vi "mxwScript_API_SetVal_NamedExternalNodeState.vi"(8 "error in (no error)":errorcluster, 10 "external node state":variant, 11 "external node name":string) -> (0 "error out":errorcluster, 3 "parameter":T1)   [LabVIEW 2020]
uses:
  codeGenAPISupport.llb/cgAPI_mxwScript_Parameter.ctl
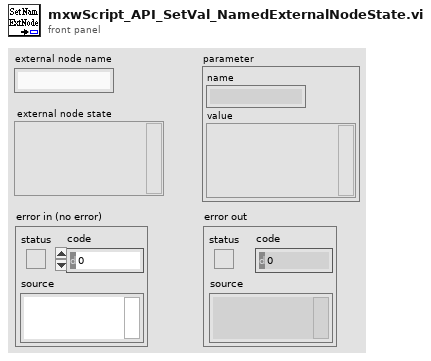
[diagram p1: front panel]
types:
  T1 = typedef "cgAPI_mxwScript_Parameter.ctl" = cluster{"name":string, "value":variant}
  T2 = cluster{"external node name":string, "external node state":variant}
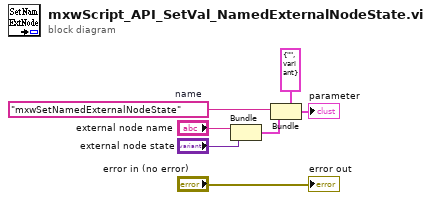
[diagram p0: block diagram]
diagram:
  w4 = "mxwSetNamedExternalNodeState"  # name
  n1 = Bundle("external node name"="external node name", "external node state"="external node state") -> (w1:T2)  [unwired: 1 out]
  n2 = Bundle(cluster=T1 {"name"="", "value"=variant} ("parameter"), "name"=w4, "value"=w1) -> (→"parameter":T1)
  "error out" <- "error in (no error)"
